vi "Random Phase HCT test.vi"() -> ()   [LabVIEW 2015]
uses:
  D:/Experiment VIs/Signal Synthesis VIs/Waveform VIs/Complex Tone VIs/CT-Params.ctl
  D:/Experiment VIs/Signal Synthesis VIs/Waveform VIs/Complex Tone VIs/CT-Phase Enum.ctl
panel:
  out "Waveform Graph":dbl[](graph)
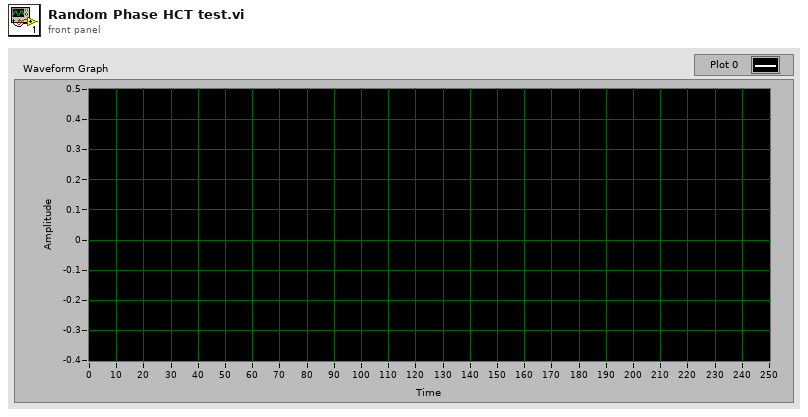
[diagram p1: front panel]
types:
  T1 = typedef "CT-Phase Enum.ctl" = enum16{"Cosine", "Random", "Alternating"}
  T2 = typedef "CT-Params.ctl" = cluster{"F0 (Hz)":dbl, "Band":cluster{"Flow (Hz)":dbl, "Fhigh (Hz)":dbl}, "Phase":T1, "Min F0 (Hz)":dbl, "Max F0 (Hz)":dbl, "ContinRandPhase":bool, "Max peak factor":dbl, "Max mod depth":dbl}
  T3 = typedef "CT-Runtime Data.ctl" = cluster{"Ncomp":i32, "MinHarm":i32, "Phase":dbl[], "Amplitude":dbl[], "Npts/frame":i32, "Last F0":dbl, "Fmin":dbl, "Fmax":dbl, "Lslope":dbl, "randphase":bool}
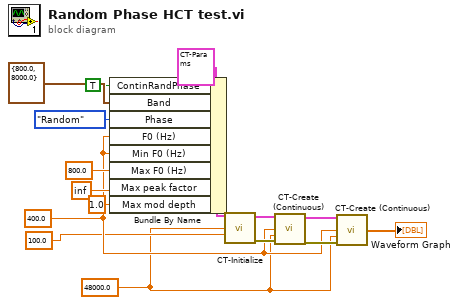
[diagram p0: block diagram]
diagram:
  w3 = 48000.0 ("Fs (Hz)")
  w5 = 400.0 ("F0 (Hz)")
  n1 = Bundle By Name(cluster=T2 {"F0 (Hz)"=0.0, "Band"={"Flow (Hz)"=0.0, "Fhigh (Hz)"=0.0}, "Phase"=enum."Cosine", "Min F0 (Hz)"=0.0, "Max F0 (Hz)"=0.0, "ContinRandPhase"=FALSE, "Max peak factor"=0.0, "Max mod depth"=0.0} ("HCT Params"), "ContinRandPhase"=TRUE, "Band"=cluster{"Flow (Hz)":dbl, "Fhigh (Hz)":dbl} {"Flow (Hz)"=800.0, "Fhigh (Hz)"=8000.0}, "Phase"=CT-Phase_Enum."Random", "F0 (Hz)"=w5, "Min F0 (Hz)"=w5, "Max F0 (Hz)"=800.0, "Max peak factor"=inf, "Max mod depth"=1.0) -> (w15:T2)
  n2 = call "CT-Initialize.vi"("HCT Params"=w15, "Fs (Hz)"=w3, "Frame size (ms)"=100.0 ("F0 (Hz)")) -> ("HCT Runtime"=w14:T3, "error out"=w13:errorcluster)  [unwired: 11 in]
  n3 = call "CT-Create (Continuous).vi"("HCT Runtime in"=w14, "F0 (Hz)"=w5, "Fs (Hz)"=w3, "error in (no error)"=w13) -> ("HCT Runtime out"=w9:T3, "error out"=w10:errorcluster)  [unwired: 9 in, 1 out]
  n4 = call "CT-Create (Continuous).vi"("HCT Runtime in"=w9, "F0 (Hz)"=w5, "Fs (Hz)"=w3, "error in (no error)"=w10) -> ("HCT"=→"Waveform Graph":dbl[])  [unwired: 9 in, 2 out]
